vi "SCMP - Generate FITS Timestamped File Paths.vi"(8 "error in":errorcluster, 9 "Camera Idx":i32, 10 "FITS Header":T2={"Wavelength (nm)"=530.15, "Exposure (s)"=0.05, "Tuning Delay (ms)"=1000.0, "Beam Type (-1/1)"=1.0, "Tuning Voltages"=[1.111, 2.222, 3.333, 4.444], "Observer"="observer", "Light Shapping Diffuser"=enum."In Beam", "Comment"="", "Data Type"=enum."HOLE", "Mod Cycles"=0, "SCD Calibration Optics"=enum."1 - Polarizer @0, I+Q", "SCD Emission Line Filter"=enum."1-557.6nm", "Cookbook"="", "COMP-S Calibration Wheel"=enum."Dark", "COMP-S Andover Filter Wheel"=enum."530.3nm/HWB 0.34nm (Fe XIV)", "FOV Rotation (deg)"=66.0, "Objective Lens Position (mm)"=0.0, "Occulter size"=0.0, "Time End"=timestamp(3382374145.421875 s since 1904-01-01), "Acc Exposure (s)"=0.0, "Time Stamp Array"=[], "Camera Serial Number"=[], "Camera Temp"=[], "Camera PI (mm)"=[], "Time Start"=timestamp(3382374145.421875 s since 1904-01-01), "Peripherals"={"ILX controler"=FALSE, "Zone temperatures"=FALSE, "Andor"=FALSE, "Andor 2"=FALSE, "PI Stages"=FALSE, "AISAS mechanisms"=FALSE, "AISAS Mech.lvclass"=refnum, "Zone temp ref"=variant, "FWs"=FALSE}, "FITS paths"=[], "Cameras"=enum."Andor", "load preset cbk"=FALSE, "periodic check count"=0, "COMP-S Calibration Wheel 2"=enum."Dark", "Calib"=enum."Dark", "Abso Aperture"=66.0, "Nominal Aperture"=66.0} {"Nominal Aperture" format="%.1f"; "Abso Aperture" format="%.1f"; "Camera PI (mm)" format="%_3g"; "Acc Exposure (s)" format="%^.3g"; "Occulter size" format="%.2f"; "Objective Lens Position (mm)" min=70.0 max=152.0 format="%.2f"; "FOV Rotation (deg)" format="%.1f"; "Exposure (s)" format="%^.3g"; "Wavelength (nm)" format="%_6g"}) -> (0 "error out":errorcluster, 2 "FITS info":T1, 3 "FITS File Path":path=path "G:/SCD Data/Level-0/20141031/20141031T094817.fits")   [LabVIEW 2014]
uses:
  Controls/SCD - FITS Cluster.ctl
  AISAS/Mech/AISAS Mech.lvclass
  AISAS/Controls/Diffuser.ctl
  Controls/FITS Data type.ctl
  Controls/SCD - Calibration Optics Filter Wheel.ctl
  Controls/SCD - EDT - Emission Line Filter Wheel.ctl
  Controls/CoMP-S Controls/Polarization Optics Filter Wheel.ctl
  Controls/CoMP-S Controls/Emission Line Filter Wheel.ctl
  AISAS/Controls/focus.ctl
  Controls/peripherals.ctl
  Controls/Cameras select.ctl
  Controls/Fits info.ctl
  Controls/Global demo.vi
  Controls/Globals.vi
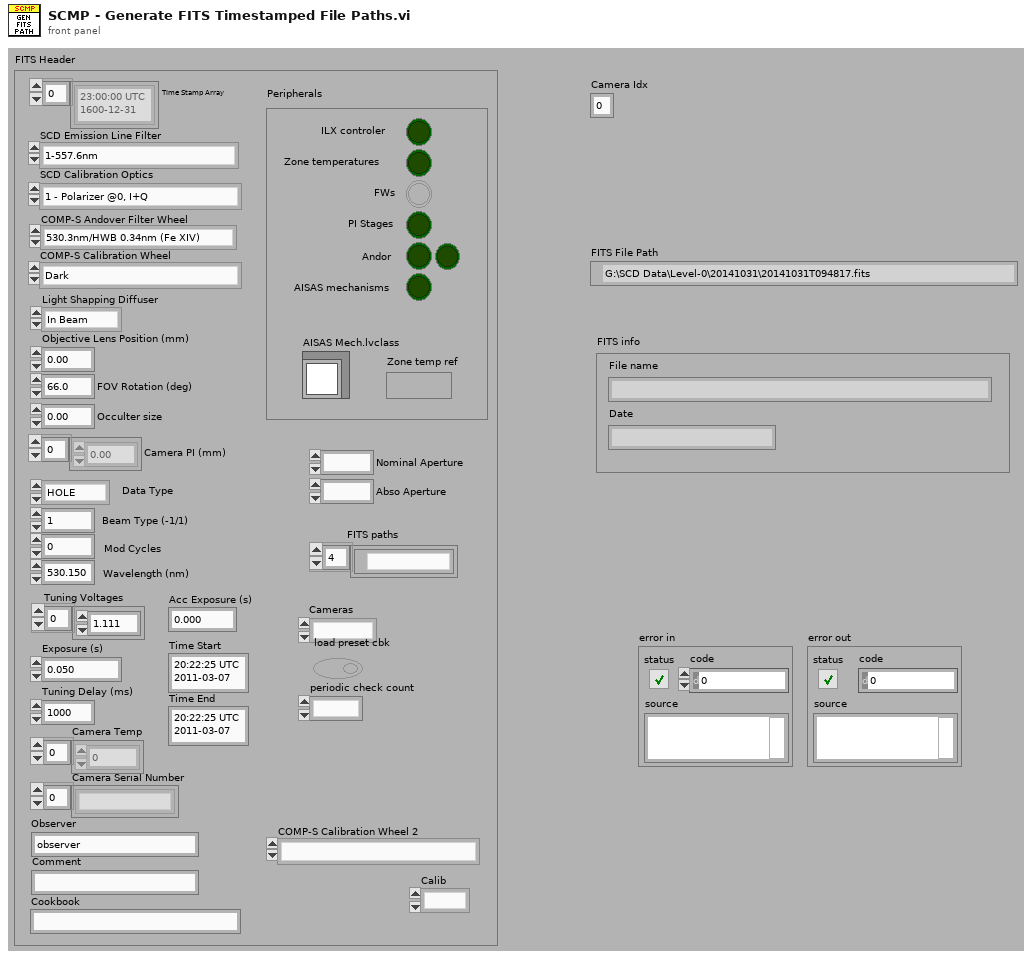
[diagram p1: front panel]
types:
  T1 = typedef "Fits info.ctl" = cluster{"File name":string, "Date":string}
  T2 = typedef "SCD - FITS Cluster.ctl" = cluster{"Wavelength (nm)":dbl, "Exposure (s)":dbl, "Tuning Delay (ms)":dbl, "Beam Type (-1/1)":dbl, "Tuning Voltages":dbl[], "Observer":string, "Light Shapping Diffuser":T3, "Comment":string, "Data Type":T4, "Mod Cycles":u16, "SCD Calibration Optics":T5, "SCD Emission Line Filter":T6, "Cookbook":string, "COMP-S Calibration Wheel":T7, "COMP-S Andover Filter Wheel":T8, "FOV Rotation (deg)":dbl, "Objective Lens Position (mm)":T9, "Occulter size":dbl, "Time End":timestamp, "Acc Exposure (s)":dbl, "Time Stamp Array":timestamp[], "Camera Serial Number":string[], "Camera Temp":dbl[], "Camera PI (mm)":dbl[], "Time Start":timestamp, "Peripherals":T10, "FITS paths":path[], "Cameras":T11, "load preset cbk":bool, "periodic check count":i32, "COMP-S Calibration Wheel 2":T7, "Calib":enum16{"Dark", "Flat"}, "Abso Aperture":dbl, "Nominal Aperture":dbl}
  T3 = typedef "Diffuser.ctl" = enum16{"Out of Beam", "In Beam"}
  T4 = typedef "FITS Data type.ctl" = enum16{"LIVE", "DARK", "FLAT", "CALI", "OBSE", "ABSO", "AURE", "TARG", "OBJE", "HOLE", "OREX", "THRO", "CHIP"}
  T5 = typedef "SCD - Calibration Optics Filter Wheel.ctl" = enum16{"1 - Polarizer @0, I+Q", "2 - Polarizer @90, I-Q", "3 - Polarizer @45, I+U", "4 - Polarizer @135, I-U", "5 - Polarizer @0, Retarder @45, I+V", "6 - Polarizer @0, Retarder @135, I-V", "7 - Dark", "8 - Clear", "9 - N/A"}
  T6 = typedef "SCD - EDT - Emission Line Filter Wheel.ctl" = enum16{"1-557.6nm", "2-587.6nm", "3-589.6nm", "4-630.2nm", "5-656.4nm", "6-849.8nm", "7-854.2nm", "8-866.2nm", "9-1083.0nm"}
  T7 = typedef "Polarization Optics Filter Wheel.ctl" = enum16{"Dark", "Clear", "Exchange Lens", "Polarizer @0, I+Q", "Polarizer @90, I-Q", "Polarizer @45, I+U", "Polarizer @135, I-U", "Polarizer @0, Retarder @45, I+V", "Polarizer @0, Retarder @135, I-V"}
  T8 = typedef "Emission Line Filter Wheel.ctl" = enum16{"530.3nm/HWB 0.34nm (Fe XIV)", "587.6nm/HBW 0.44nm (He I D3)", "637.5nm/HBW 0.53nm (Fe X)", "656.3nm/HBW 0.57nm (H-Alpha)", "789.2nm/HBW 0.85nm (Fe XI)", "854.2nm/HBW 1.01nm (Ca I)", "1074.7nm/HBW 2.34nm (Fe XIII)", "1079.8nm/HBW 1.64nm (Fe XIII)", "1083.0nm/HBW 1.66nm (He I)"}
  T9 = typedef "focus.ctl" = dbl
  T10 = typedef "peripherals.ctl" = cluster{"ILX controler":bool, "Zone temperatures":bool, "Andor":bool, "Andor 2":bool, "PI Stages":bool, "AISAS mechanisms":bool, "AISAS Mech.lvclass":refnum<class "AISAS Mech.lvclass">, "Zone temp ref":variant, "FWs":bool}
  T11 = typedef "Cameras select.ctl" = enum16{"Andor", "GDR"}
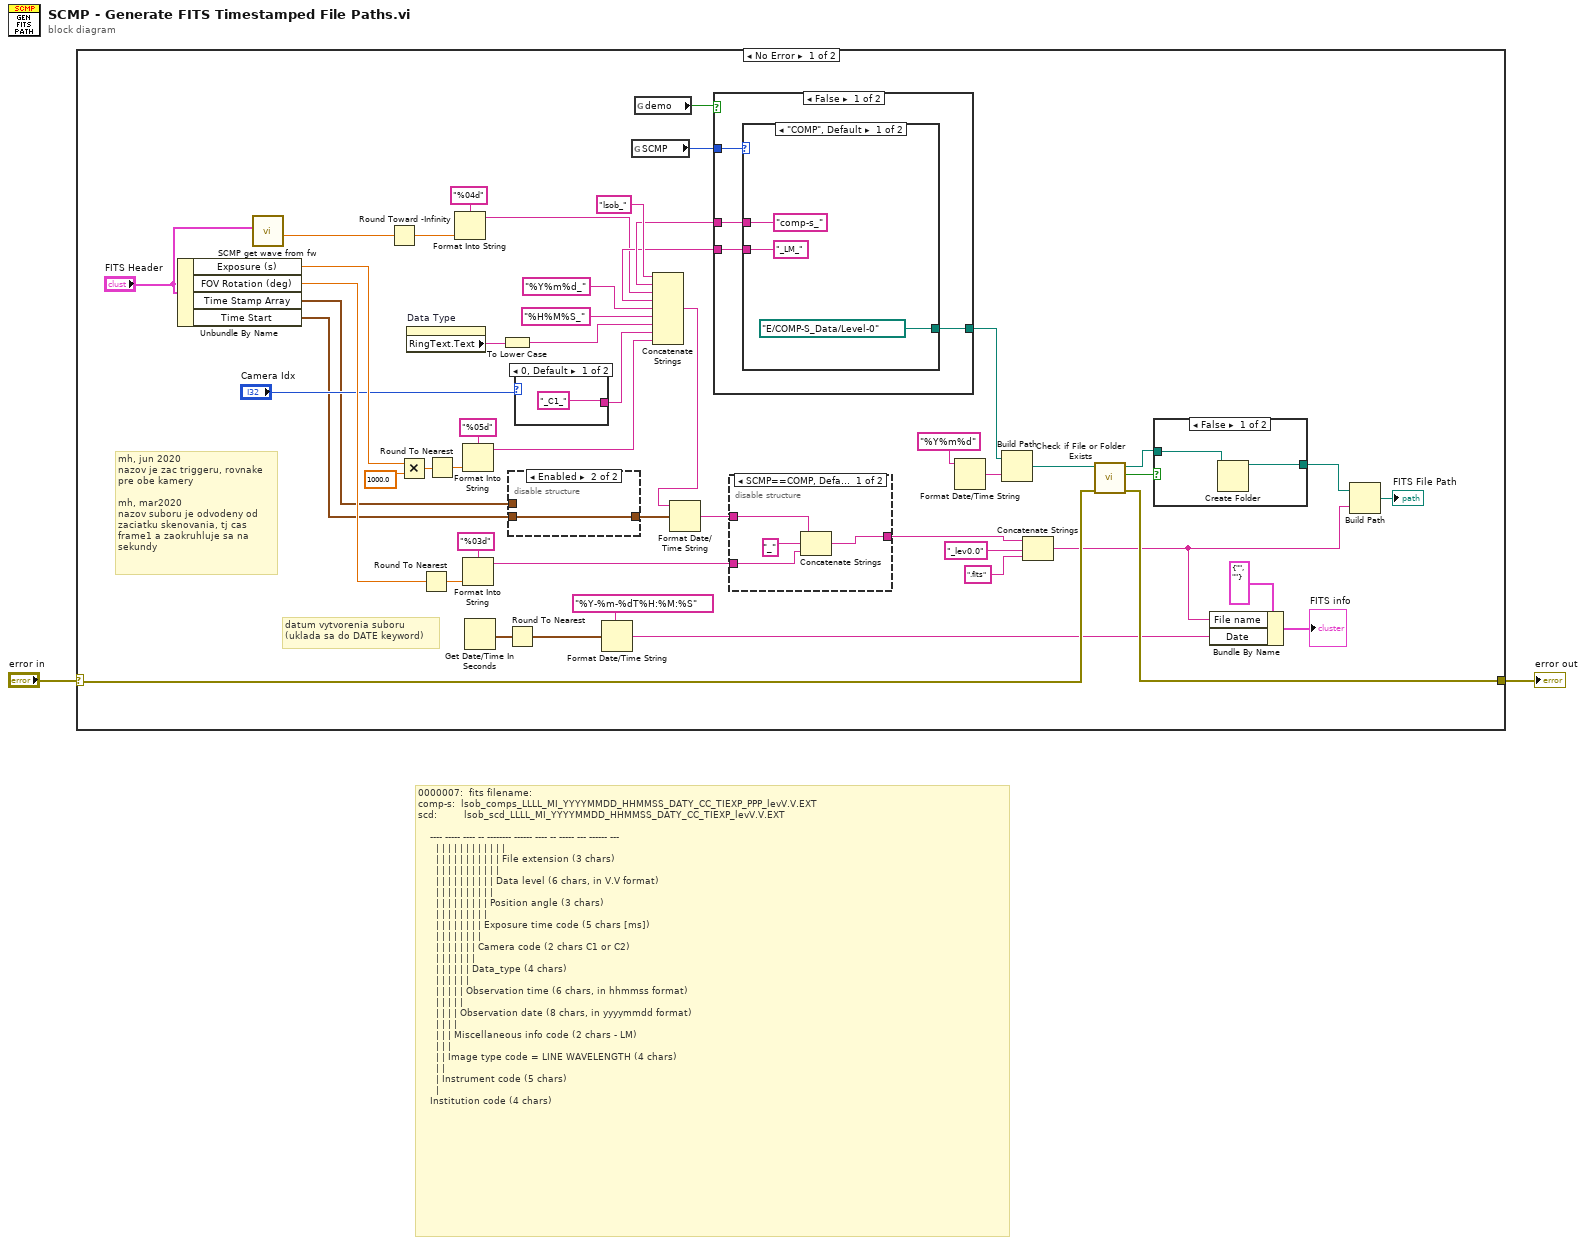
[diagram p0: block diagram]
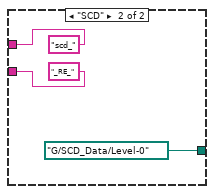
[diagram p2: hidden frame]
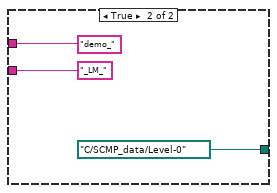
[diagram p3: hidden frame]
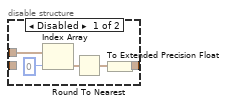
[diagram p4: hidden frame]
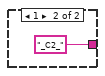
[diagram p5: hidden frame]
diagram:
  # "0000007:  fits filename:\ncomp-s:  lsob_comps_LLLL_MI_YYYYMMDD_HHMMSS_DATY_CC_TIEXP_PPP_levV.V.EXT\nscd:         lsob_scd_LLLL_MI_YYYYMMDD_HHMMSS_DATY_CC_TIEXP_levV.V.EXT\n\n    ---- ----- ---- -- -------- ------ ---- -- ----- --- ------ ---\n      | | | | | | | | | | | |\n      | | | | | | | | | | | File extension (3 chars)\n      | | | | | | | | | | |\n      | | | | | | | | | | Data level (6 chars, in V.V format)\n      | | | | | | | | | |\n      | | | | | | | | | Position angle (3 chars)\n      | | | | | | | | |\n      | | | | | | | | Exposure time code (5 chars [ms])\n      | | | | | | | |\n      | | | | | | | Camera code (2 chars C1 or C2)\n      | | | | | | |\n      | | | | | | Data_type (4 chars)\n      | | | | | |\n      | | | | | Observation time (6 chars, in hhmmss format)\n      | | | | |\n      | | | | Observation date (8 chars, in yyyymmdd format)\n      | | | |\n      | | | Miscellaneous info code (2 chars - LM)\n      | | |\n      | | Image type code = LINE WAVELENGTH (4 chars)\n      | |\n      | Instrument code (5 chars)\n      |\n    Institution code (4 chars)"
  n1 = case shown="No Error" "error in" {
    selector: "error in" -> [w43 w82]
    tunnel: [w42 w82] -> w2
    frame No Error {
      # "datum vytvorenia suboru\n(uklada sa do DATE keyword)"
      # "mh, jun 2020\nnazov je zac triggeru, rovnake pre obe kamery\n\nmh, mar2020\nnazov suboru je odvodeny od zaciatku skenovania, tj cas frame1 a zaokruhluje sa na sekundy"
      n2 = Unbundle By Name("FITS Header") -> ("Exposure (s)"=w24:dbl, "FOV Rotation (deg)"=w22:dbl, "Time Stamp Array"=w10:timestamp[], "Time Start"=w7:timestamp)
      n3 = call "SCMP get wave from fw.vi"("FITS Header"="FITS Header") -> ("value"=w3:dbl)  [unwired: 9 in, 1 out]
      n4 = Round Toward -Infinity(1:w3) -> (0:w34:dbl)
      n5 = Multiply(x=w24, y=1000.0) -> (x*y=w31:dbl)
      n6 = property on="Data Type" class="Enum (strict)"() -> ("RingText.Text"=w13:string)  [unwired: 2 in, 2 out]
      n7 = Round To Nearest(number=w22) -> (nearest integer value=w20:dbl)
      n8 = Round To Nearest(number=w31) -> (nearest integer value=w30:dbl)
      n9 = Format Into String(format string="%04d", w34) -> (resulting string=w33:string)  [unwired: 2 in, 1 out]
      n10 = Format Into String(format string="%05d", w30) -> (resulting string=w27:string)  [unwired: 2 in, 1 out]
      n11 = Format Into String(format string="%03d", w20) -> (resulting string=w19:string)  [unwired: 2 in, 1 out]
      n12 = Get Date/Time In Seconds() -> (seconds since 1Jan1904=w8:timestamp)
      n13 = To Lower Case(string=w13) -> (all lower case string=w23:string)
      n14 = Round To Nearest(number=w8) -> (nearest integer value=w9:timestamp)
      n15 = disable-structure shown="Enabled" {
        disable-tunnel: [w69 w71] -> w11
        disable-tunnel: w10 -> [w68 _]
        disable-tunnel: w7 -> [_ w71]
        frame Disabled {
          n16 = Index Array(array=w68, index=0) -> (element=w67:timestamp)
          n17 = Round To Nearest(number=w67) -> (nearest integer value=w69:timestamp)
          n18 = To Extended Precision Float(1:w69) -> ()  [unwired: 1 out]
        }
        frame Enabled {
        }
      }
      n19 = case shown="0, Default" "Camera Idx" {
        tunnel: ["_C1_" ("time format string (%c)") "_C2_" ("time format string (%c)")] -> w28
        frame 0, Default {
        }
        frame 1 {
        }
      }
      n20 = Format Date/Time String(time format string (%c)="%Y-%m-%dT%H:%M:%S", seconds (now)=w9) -> (date/time string=w15:string)  [unwired: 1 in]
      n21 = global read "Globals.vi" "SCMP"() -> (w5:enum16{"COMP", "SCD"})
      n22 = global read "Global demo.vi" "demo"() -> (w6:bool)
      n23 = case shown="False" w6 {
        tunnel: [w57 path "C:/SCMP_data/Level-0" ("SCMP demo Base Path")] -> w53
        tunnel: [w56 "demo_" ("string")] -> w40
        tunnel: [w55 "_LM_" ("string")] -> w39
        tunnel: w5 -> [w54 _]
        frame False {
          n24 = case shown="\"COMP\", Default" w54 {
            tunnel: [path "E:/COMP-S_Data/Level-0" ("COMPs Base Path") path "G:/SCD_Data/Level-0" ("SCD Base Path")] -> w57
            tunnel: ["comp-s_" ("string") "scd_" ("string")] -> w56
            tunnel: ["_LM_" ("string") "_RE_" ("string")] -> w55
            frame "COMP", Default {
            }
            frame "SCD" {
            }
          }
        }
        frame True {
        }
      }
      n25 = Concatenate Strings("lsob_" ("string"), w40, w33, w39, "%Y%m%d_" ("time format string (%c)"), "%H%M%S_" ("time format string (%c)"), w23, w28, w27) -> (w45:string)
      n26 = Format Date/Time String(time format string (%c)=w45, seconds (now)=w11) -> (date/time string=w29:string)  [unwired: 1 in]
      n27 = disable-structure shown="SCMP==COMP, Default" {
        disable-tunnel: w29 -> [w77 w78]
        disable-tunnel: [w75 w78] -> w25
        disable-tunnel: w19 -> [w74 _]
        frame condition #0 (active) {
          n28 = Concatenate Strings(w77, "_" ("string"), w74) -> (w75:string)
        }
        frame condition #1 {
        }
      }
      n29 = Format Date/Time String(time format string (%c)="%Y%m%d") -> (date/time string=w50:string)  [unwired: 2 out]
      n30 = Build Path(base path=w53, name or relative path=w50) -> (appended path=w52:path)
      n31 = Concatenate Strings(w25, "_lev0.0" ("string"), ".fits" ("string")) -> (w14:string)
      n32 = call <vilib>:"Check if File or Folder Exists.vi"("error in (no error)"=w43, "path"=w52) -> ("error out"=w42:errorcluster, "file or folder exists?"=w47:bool, "dup path"=w51:path)  [unwired: 7 out]
      n33 = case shown="False" w47 {
        tunnel: [w80 w81] -> w46
        tunnel: w51 -> [w79 w81]
        frame False {
          n34 = Create Folder(path (use dialog)=w79) -> (created path=w80:path)  [unwired: 1 in, 3 out]
        }
        frame True {
        }
      }
      n35 = Bundle By Name(cluster=cluster{"File name":string, "Date":string} {"File name"="", "Date"=""} ("FITS info"), "File name"=w14, "Date"=w15) -> (→"FITS info":cluster{"File name":string, "Date":string})
      n36 = Build Path(base path=w46, name or relative path=w14) -> (appended path=→"FITS File Path":path)
    }
    frame Error {
    }
  }
  "error out" <- w2
